vi "Read XboxJoysticks.vi"(8 "error in (no error)":errorcluster, 11 "XBoxController in":refnum<class "XBoxController.lvclass">) -> (0 "error out":errorcluster, 2 "XboxJoysticks":T1 {"RightJoystick"."Right" scale=-1.0..1.0; "RightJoystick"."Forward" scale=-1.0..1.0; "LeftJoystick"."Right" scale=-1.0..1.0; "LeftJoystick"."Forward" scale=-1.0..1.0}, 3 "XBoxController out":refnum<class "XBoxController.lvclass">)   [LabVIEW 2013, in "XBoxController.lvclass"]
uses:
  XBoxController.lvclass
  XBoxController.lvclass/XBoxController.ctl
panel:
  in  "Deadband":dbl(knob)=0.2 step=0.01 scale=0.0..0.5
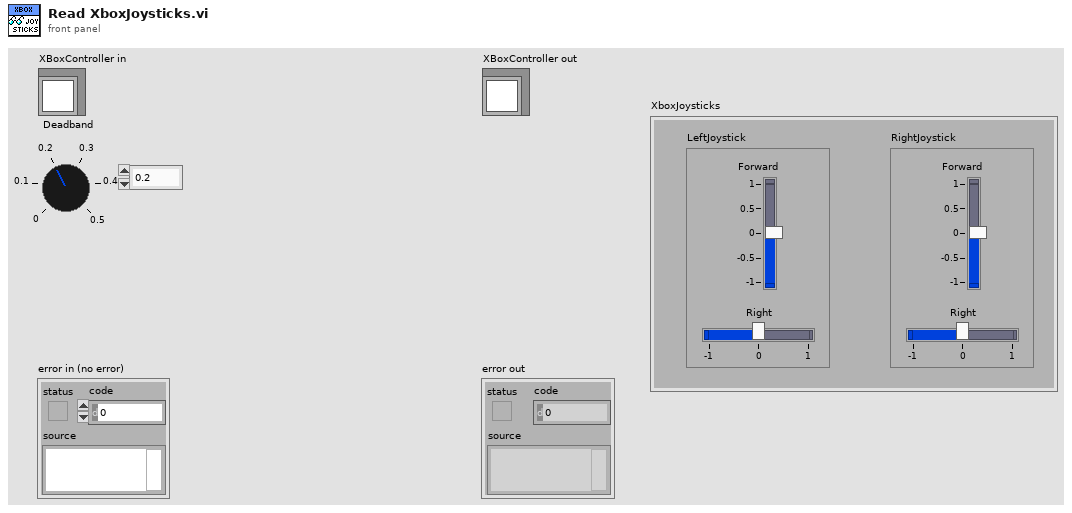
[diagram p1: front panel]
types:
  T1 = cluster{"LeftJoystick":cluster{"Forward":dbl, "Right":dbl}, "RightJoystick":cluster{"Forward":dbl, "Right":dbl}}
  T2 = typedef "WPI_JoystickDevRef.ctl" = cluster{"Device":T3}
  T3 = typedef "WPI_JoystickDeviceEnum.ctl" = enum16{"USB 1", "USB 2", "USB 3", "USB 4", "Kinect 1", "Kinect 2"}
  T4 = cluster{"axis 1 (x)":dbl, "axis 2 (y)":dbl, "axis 3 (throttle)":dbl, "axis 4":dbl, "axis 5":dbl, "axis 6":dbl}
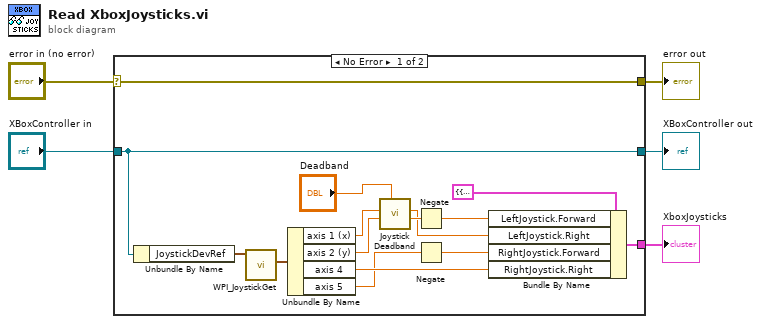
[diagram p0: block diagram]
diagram:
  n1 = case shown="No Error" "error in (no error)" {
    selector: "error in (no error)" -> [w20 w21]
    tunnel: [w20 w21] -> w4
    tunnel: [w11 w22] -> w2
    tunnel: "XBoxController in" -> [w11 w22]
    tunnel: [w16 _] -> w1
    frame No Error {
      n2 = Unbundle By Name(w11) -> ("JoystickDevRef"=w19:T2)
      n3 = call <vilib>:"WPI_JoystickGet.vi"("JoystickDevRef"=w19) -> ("Axes"=w18:T4)  [unwired: 4 in, 2 out]
      n4 = Unbundle By Name(w18) -> ("axis 1 (x)"=w10:dbl, "axis 2 (y)"=w7:dbl, "axis 4"=w15:dbl, "axis 5"=w14:dbl)
      n5 = call "Joystick Deadband.vi"("Deadband"="Deadband", "Y in"=w7, "X in"=w10) -> ("Y out"=w8:dbl, "X out"=w6:dbl)  [unwired: 7 in]
      n6 = Negate(x=w8) -> (-x=w13:dbl)
      n7 = Negate(x=w14) -> (-x=w12:dbl)
      n8 = Bundle By Name(cluster=T1 {"LeftJoystick"={"Forward"=0.0, "Right"=0.0}, "RightJoystick"={"Forward"=0.0, "Right"=0.0}} ("XboxJoysticks"), "LeftJoystick.Forward"=w13, "LeftJoystick.Right"=w6, "RightJoystick.Forward"=w12, "RightJoystick.Right"=w15) -> (w16:T1)
    }
    frame Error {
    }
  }
  "error out" <- w4
  "XBoxController out" <- w2
  "XboxJoysticks" <- w1
